vi "Main.vi"() -> ()   [LabVIEW 2018] (continued)
                    n939 = Delete From Array(array=w5529, length=2 ("长度"), index=0 ("索引")) -> (deleted portion=w5517:string[], array with subset deleted=w5526:string[])
                    n940 = call "SQL_Update.vi"("查询语句"=w5514, "表名"="Online", "error in (no error)"=w5522, "列名对应的值"=w5517, "列名"=string[] ["Last_Station", "Last_Result"], "connection reference"=w5523) -> ("error out"=w5521:errorcluster, "connection reference 2"=w5520:T5)  [unwired: 4 in]
                    n941 = call "SQL_Update.vi"("查询语句"=w5514, "表名"="Rework", "error in (no error)"=w5521, "列名对应的值"=w5526, "列名"=string[] ["ST401_Date", "ST401_Time", "ST401_Result", "ST401_PanelNumber", "ST401_Shield"], "connection reference"=w5520) -> ("error out"=w5515:errorcluster)  [unwired: 4 in, 1 out]
                    n942 = Unbundle By Name(w5515) -> ("status"=w5532:bool)
                    n943 = Equal?(x="", y=w5524) -> (x = y?=w5531:bool)
                    n944 = Or(x=w5532, y=w5531) -> (x .or. y?=w5530:bool)
                    n945 = case shown="真" w5530 {
                      tunnel: ["1" ("数据保存请求回复") "2" ("数据保存请求回复")] -> w5516
                      frame False {
                      }
                      frame True {
                      }
                    }
                  }
                }
              }
            }
            "数据保存请求回复401" <- w5445
            n946 = local write "401数据回复写入"(w5444) -> ()
            n947 = Delete From Array(array=w5433, length=2 ("长度"), index=0 ("索引")) -> (array with subset deleted=w5440:string[])  [unwired: 1 out]
            n948 = Insert Into Array(array=w5440, index=2 ("索引"), new element=w5432) -> (w5439:string[])
            n949 = Insert Into Array(array=string[][] [] ("数组"), index (row)=0 ("索引 (行)"), new element=w5439) -> (w5441:string[][])  [unwired: 1 in]
            n950 = Transpose 2D Array(2D array=w5441) -> (transposed array=w5431:string[][])
            n951 = property on="ST401_DATA" class="MCListbox (严格)"("ItemNames"=w5431) -> ()  [unwired: 2 in, 2 out]
            "ST401数据读取（事件）" <- FALSE ("ST401数据保存请求（事件）")
          }
          event "ST402扫码请求（事件）": Value Change {
            n952 = event-data() -> ()  [unwired: 1 in, 2 out]
            n953 = local read "402二维码"() -> (w5540:string)
            n954 = Concatenate Strings("Where QRCode='" ("查询语句"), w5540, "'" ("字符串")) -> (w5549:string)
            n955 = call "SQL_Select.vi"("要读取的列名"=string[] ["Last_Station", "Last_Result"], "表名"="Online", "error in (no error)"=w5541, "查询语句"=w5549, "查询条件"=TRUE, "connection reference"=w5542) -> ("error out"=w5539:errorcluster, "数据"=w5548:string[][])  [unwired: 3 in, 1 out]
            n956 = case shown="无错误" w5539 {
              tunnel: w5548 -> [w5558 _]
              tunnel: ["1" ("右扫码请求回复") "2" ("右扫码请求回复")] -> w5538
              tunnel: [TRUE TRUE] -> w5537
              frame No Error {
                n957 = Index Array(array=w5558, index (row)=0 ("索引 (行)")) -> (element=w5555:string[])  [unwired: 1 in]
                n958 = Index Array(array=w5555, index #1=0 ("索引 (行)")) -> (element #1=→"上一站号 (402)":string, element #2=→"上一站结果 (402)":string)  [unwired: 1 in]
              }
              frame Error {
              }
            }
            "扫码请求回复402" <- w5538
            n959 = local write "402扫码回复写入"(w5537) -> ()
            "ST402扫码请求（事件）" <- FALSE ("ST402扫码请求（事件）")
          }
          event "ST402数据读取（事件）": Value Change {
            w5583 = 0 ("索引 (行)")
            n960 = event-data() -> ()  [unwired: 1 in, 2 out]
            n961 = local read "402二维码"() -> (w5562:string)
            n962 = Concatenate Strings("Where QRCode='" ("查询语句"), w5562, "'" ("字符串")) -> (w5590:string)
            n963 = call "SQL_Select.vi"("要读取的列名"=string[] ["Rework_Status"], "表名"="Online", "error in (no error)"=w5576, "查询语句"=w5590, "查询条件"=TRUE, "connection reference"=w5577) -> ("error out"=w5585:errorcluster, "数据"=w5589:string[][], "connection reference out"=w5586:T5)  [unwired: 3 in]
            n964 = Index Array(array=w5589, index (row)=w5583, index (col)=w5583) -> (element=w5588:string)
            n965 = Equal?(x=w5588, y="T") -> (x = y?=w5587:bool)
            n966 = local read "402data"() -> (w5563:string[])
            n967 = case shown="真" w5587 {
              tunnel: [w5604 w5610] -> w5575
              tunnel: w5563 -> [w5603 w5613]
              tunnel: [w5598 w5609] -> w5573
              tunnel: w5562 -> [w5597 w5612]
              tunnel: w5590 -> [w5596 w5611]
              tunnel: w5586 -> [w5595 w5624]
              tunnel: w5585 -> [w5594 w5623]
              tunnel: [TRUE w5608] -> w5574
              frame False {
                n968 = call "SQL_Update.vi"("查询语句"=w5596, "表名"="Online", "error in (no error)"=w5594, "列名对应的值"=w5603, "列名"=string[] ["Last_Station", "Last_Result", "ST402_Date", "ST402_Time", "ST402_Result", "ST402_PanelNumber", "ST402_Shield"], "connection reference"=w5595) -> ("error out"=w5598:errorcluster)  [unwired: 4 in, 1 out]
                n969 = Unbundle By Name(w5598) -> ("status"=w5602:bool)
                n970 = Equal?(x=w5597, y="") -> (x = y?=w5600:bool)
                n971 = Or(x=w5602, y=w5600) -> (x .or. y?=w5599:bool)
                n972 = case shown="假" w5599 {
                  tunnel: ["1" ("数据保存请求回复") "2" ("数据保存请求回复")] -> w5604
                  frame False {
                  }
                  frame True {
                  }
                }
              }
              frame True {
                w5619 = 0 ("索引 (行)")
                n973 = call "SQL_Select.vi"("要读取的列名"=string[] ["[402]"], "表名"="Rework_List", "error in (no error)"=w5623, "查询语句"=w5611, "查询条件"=TRUE, "connection reference"=w5624) -> ("error out"=w5614:errorcluster, "数据"=w5620:string[][], "connection reference out"=w5615:T5)  [unwired: 3 in]
                n974 = Index Array(array=w5620, index (row)=w5619, index (col)=w5619) -> (element=w5618:string)
                n975 = Equal?(x=w5618, y="T") -> (x = y?=w5616:bool)
                n976 = case shown="真" w5616 {
                  tunnel: w5615 -> [w5633 w5653]
                  tunnel: w5614 -> [w5634 w5652]
                  tunnel: w5613 -> [w5632 w5659]
                  tunnel: w5612 -> [w5629 w5654]
                  tunnel: w5611 -> [w5631 w5644]
                  tunnel: [w5628 w5646] -> w5610
                  tunnel: [w5630 w5645] -> w5609
                  tunnel: [TRUE TRUE] -> w5608
                  frame False {
                    n977 = call "SQL_Update.vi"("查询语句"=w5631, "表名"="Online", "error in (no error)"=w5634, "列名对应的值"=w5632, "列名"=string[] ["Last_Station", "Last_Result", "ST402_Date", "ST402_Time", "ST402_Result", "ST402_PanelNumber", "ST402_Shield"], "connection reference"=w5633) -> ("error out"=w5630:errorcluster)  [unwired: 4 in, 1 out]
                    n978 = Unbundle By Name(w5630) -> ("status"=w5638:bool)
                    n979 = Equal?(x=w5629, y="") -> (x = y?=w5636:bool)
                    n980 = Or(x=w5638, y=w5636) -> (x .or. y?=w5635:bool)
                    n981 = case shown="假" w5635 {
                      tunnel: ["1" ("数据保存请求回复") "2" ("数据保存请求回复")] -> w5628
                      frame False {
                      }
                      frame True {
                      }
                    }
                  }
                  frame True {
                    n982 = Delete From Array(array=w5659, length=2 ("长度"), index=0 ("索引")) -> (deleted portion=w5647:string[], array with subset deleted=w5656:string[])
                    n983 = call "SQL_Update.vi"("查询语句"=w5644, "表名"="Online", "error in (no error)"=w5652, "列名对应的值"=w5647, "列名"=string[] ["Last_Station", "Last_Result"], "connection reference"=w5653) -> ("error out"=w5651:errorcluster, "connection reference 2"=w5650:T5)  [unwired: 4 in]
                    n984 = call "SQL_Update.vi"("查询语句"=w5644, "表名"="Rework", "error in (no error)"=w5651, "列名对应的值"=w5656, "列名"=string[] ["ST402_Date", "ST402_Time", "ST402_Result", "ST402_PanelNumber", "ST402_Shield"], "connection reference"=w5650) -> ("error out"=w5645:errorcluster)  [unwired: 4 in, 1 out]
                    n985 = Unbundle By Name(w5645) -> ("status"=w5662:bool)
                    n986 = Equal?(x="", y=w5654) -> (x = y?=w5661:bool)
                    n987 = Or(x=w5662, y=w5661) -> (x .or. y?=w5660:bool)
                    n988 = case shown="真" w5660 {
                      tunnel: ["1" ("数据保存请求回复") "2" ("数据保存请求回复")] -> w5646
                      frame False {
                      }
                      frame True {
                      }
                    }
                  }
                }
              }
            }
            "数据保存请求回复402" <- w5575
            n989 = local write "402数据回复写入"(w5574) -> ()
            n990 = Delete From Array(array=w5563, length=2 ("长度"), index=0 ("索引")) -> (array with subset deleted=w5570:string[])  [unwired: 1 out]
            n991 = Insert Into Array(array=w5570, index=2 ("索引"), new element=w5562) -> (w5569:string[])
            n992 = Insert Into Array(array=string[][] [] ("数组"), index (row)=0 ("索引 (行)"), new element=w5569) -> (w5571:string[][])  [unwired: 1 in]
            n993 = Transpose 2D Array(2D array=w5571) -> (transposed array=w5561:string[][])
            n994 = property on="ST402_DATA" class="MCListbox (严格)"("ItemNames"=w5561) -> ()  [unwired: 2 in, 2 out]
            "ST402数据读取（事件）" <- FALSE ("ST402数据保存请求（事件）")
          }
          event "ST501扫码请求（事件）": Value Change {
            n995 = event-data() -> ()  [unwired: 1 in, 2 out]
            n996 = local read "501二维码"() -> (w5669:string)
            n997 = Concatenate Strings("Where QRCode='" ("查询语句"), w5669, "'" ("字符串")) -> (w5679:string)
            n998 = call "SQL_Select.vi"("要读取的列名"=string[] ["Last_Station", "Last_Result"], "表名"="Online", "error in (no error)"=w5671, "查询语句"=w5679, "查询条件"=TRUE, "connection reference"=w5672) -> ("error out"=w5670:errorcluster, "数据"=w5678:string[][])  [unwired: 3 in, 1 out]
            n999 = case shown="无错误" w5670 {
              tunnel: w5678 -> [w5688 _]
              tunnel: ["1" ("右扫码请求回复") "2" ("右扫码请求回复")] -> w5668
              tunnel: [TRUE TRUE] -> w5667
              frame No Error {
                n1000 = Index Array(array=w5688, index (row)=0 ("索引 (行)")) -> (element=w5685:string[])  [unwired: 1 in]
                n1001 = Index Array(array=w5685, index #1=0 ("索引 (行)")) -> (element #1=→"上一站号 (501)":string, element #2=→"上一站结果 (501)":string)  [unwired: 1 in]
              }
              frame Error {
              }
            }
            "扫码请求回复501" <- w5668
            n1002 = local write "501扫码回复输入"(w5667) -> ()
            "ST501扫码请求（事件）" <- FALSE ("ST501扫码请求（事件）")
          }
          event "ST501数据读取（事件）": Value Change {
            w5713 = 0 ("索引 (行)")
            n1003 = event-data() -> ()  [unwired: 1 in, 2 out]
            n1004 = local read "501二维码"() -> (w5692:string)
            n1005 = Concatenate Strings("Where QRCode='" ("查询语句"), w5692, "'" ("字符串")) -> (w5720:string)
            n1006 = call "SQL_Select.vi"("要读取的列名"=string[] ["Rework_Status"], "表名"="Online", "error in (no error)"=w5706, "查询语句"=w5720, "查询条件"=TRUE, "connection reference"=w5707) -> ("error out"=w5715:errorcluster, "数据"=w5719:string[][], "connection reference out"=w5716:T5)  [unwired: 3 in]
            n1007 = Index Array(array=w5719, index (row)=w5713, index (col)=w5713) -> (element=w5718:string)
            n1008 = Equal?(x=w5718, y="T") -> (x = y?=w5717:bool)
            n1009 = local read "501data"() -> (w5693:string[])
            n1010 = case shown="真" w5717 {
              tunnel: [w5734 w5740] -> w5704
              tunnel: w5693 -> [w5733 w5743]
              tunnel: [w5728 w5739] -> w5703
              tunnel: w5692 -> [w5727 w5742]
              tunnel: w5720 -> [w5726 w5741]
              tunnel: w5716 -> [w5725 w5754]
              tunnel: w5715 -> [w5724 w5753]
              tunnel: [TRUE w5738] -> w5705
              frame False {
                n1011 = call "SQL_Update.vi"("查询语句"=w5726, "表名"="Online", "error in (no error)"=w5724, "列名对应的值"=w5733, "列名"=string[] ["Last_Station", "Last_Result", "ST501_Date", "ST501_Time", "ST501_Result", "ST501_PanelNumber", "ST501_Shield"], "connection reference"=w5725) -> ("error out"=w5728:errorcluster)  [unwired: 4 in, 1 out]
                n1012 = Unbundle By Name(w5728) -> ("status"=w5732:bool)
                n1013 = Equal?(x=w5727, y="") -> (x = y?=w5730:bool)
                n1014 = Or(x=w5732, y=w5730) -> (x .or. y?=w5729:bool)
                n1015 = case shown="假" w5729 {
                  tunnel: ["1" ("数据保存请求回复") "2" ("数据保存请求回复")] -> w5734
                  frame False {
                  }
                  frame True {
                  }
                }
              }
              frame True {
                w5749 = 0 ("索引 (行)")
                n1016 = call "SQL_Select.vi"("要读取的列名"=string[] ["[501]"], "表名"="Rework_List", "error in (no error)"=w5753, "查询语句"=w5741, "查询条件"=TRUE, "connection reference"=w5754) -> ("error out"=w5744:errorcluster, "数据"=w5750:string[][], "connection reference out"=w5745:T5)  [unwired: 3 in]
                n1017 = Index Array(array=w5750, index (row)=w5749, index (col)=w5749) -> (element=w5748:string)
                n1018 = Equal?(x=w5748, y="T") -> (x = y?=w5746:bool)
                n1019 = case shown="真" w5746 {
                  tunnel: w5745 -> [w5763 w5783]
                  tunnel: w5744 -> [w5764 w5782]
                  tunnel: w5743 -> [w5762 w5789]
                  tunnel: w5742 -> [w5759 w5784]
                  tunnel: w5741 -> [w5761 w5774]
                  tunnel: [w5758 w5776] -> w5740
                  tunnel: [w5760 w5775] -> w5739
                  tunnel: [TRUE TRUE] -> w5738
                  frame False {
                    n1020 = call "SQL_Update.vi"("查询语句"=w5761, "表名"="Online", "error in (no error)"=w5764, "列名对应的值"=w5762, "列名"=string[] ["Last_Station", "Last_Result", "ST501_Date", "ST501_Time", "ST501_Result", "ST501_PanelNumber", "ST501_Shield"], "connection reference"=w5763) -> ("error out"=w5760:errorcluster)  [unwired: 4 in, 1 out]
                    n1021 = Unbundle By Name(w5760) -> ("status"=w5768:bool)
                    n1022 = Equal?(x=w5759, y="") -> (x = y?=w5766:bool)
                    n1023 = Or(x=w5768, y=w5766) -> (x .or. y?=w5765:bool)
                    n1024 = case shown="假" w5765 {
                      tunnel: ["1" ("数据保存请求回复") "2" ("数据保存请求回复")] -> w5758
                      frame False {
                      }
                      frame True {
                      }
                    }
                  }
                  frame True {
                    n1025 = Delete From Array(array=w5789, length=2 ("长度"), index=0 ("索引")) -> (deleted portion=w5777:string[], array with subset deleted=w5786:string[])
                    n1026 = call "SQL_Update.vi"("查询语句"=w5774, "表名"="Online", "error in (no error)"=w5782, "列名对应的值"=w5777, "列名"=string[] ["Last_Station", "Last_Result"], "connection reference"=w5783) -> ("error out"=w5781:errorcluster, "connection reference 2"=w5780:T5)  [unwired: 4 in]
                    n1027 = call "SQL_Update.vi"("查询语句"=w5774, "表名"="Rework", "error in (no error)"=w5781, "列名对应的值"=w5786, "列名"=string[] ["ST501_Date", "ST501_Time", "ST501_Result", "ST501_PanelNumber", "ST501_Shield"], "connection reference"=w5780) -> ("error out"=w5775:errorcluster)  [unwired: 4 in, 1 out]
                    n1028 = Unbundle By Name(w5775) -> ("status"=w5792:bool)
                    n1029 = Equal?(x="", y=w5784) -> (x = y?=w5791:bool)
                    n1030 = Or(x=w5792, y=w5791) -> (x .or. y?=w5790:bool)
                    n1031 = case shown="真" w5790 {
                      tunnel: ["1" ("数据保存请求回复") "2" ("数据保存请求回复")] -> w5776
                      frame False {
                      }
                      frame True {
                      }
                    }
                  }
                }
              }
            }
            "数据保存请求回复501" <- w5704
            n1032 = local write "501数据回复输入"(w5705) -> ()
            n1033 = Delete From Array(array=w5693, length=2 ("长度"), index=0 ("索引")) -> (array with subset deleted=w5700:string[])  [unwired: 1 out]
            n1034 = Insert Into Array(array=w5700, index=2 ("索引"), new element=w5692) -> (w5699:string[])
            n1035 = Insert Into Array(array=string[][] [] ("数组"), index (row)=0 ("索引 (行)"), new element=w5699) -> (w5701:string[][])  [unwired: 1 in]
            n1036 = Transpose 2D Array(2D array=w5701) -> (transposed array=w5691:string[][])
            n1037 = property on="ST501_DATA" class="MCListbox (严格)"("ItemNames"=w5691) -> ()  [unwired: 2 in, 2 out]
            "ST501数据读取（事件）" <- FALSE ("ST501数据读取（事件）")
          }
          event "ST502扫码请求（事件）": Value Change {
            w5797 = path "D:/op50" ("路径")
            n1038 = event-data() -> ()  [unwired: 1 in, 2 out]
            n1039 = List Folder(path=w5797) -> (filenames=w5796:string[])  [unwired: 3 in, 3 out]
            n1040 = for {
              tunnel: w5796 -> [w5815] mode=indexing
              tunnel: w5797 -> [w5816]
              n1041 = Build Path(base path=w5816, name or relative path=w5815) -> (appended path=w5813:path)
              n1042 = Delete(path (use dialog)=w5813, entire hierarchy (F)=TRUE ("整个层次结构(F)")) -> ()  [unwired: 3 in, 3 out]
            }
            n1043 = local read "502二维码"() -> (w5802:string)
            n1044 = Concatenate Strings("Where QRCode='" ("查询语句"), w5802, "'" ("字符串")) -> (w5811:string)
            n1045 = call "SQL_Select.vi"("要读取的列名"=string[] ["Last_Station", "Last_Result"], "表名"="Online", "error in (no error)"=w5803, "查询语句"=w5811, "查询条件"=TRUE, "connection reference"=w5804) -> ("error out"=w5801:errorcluster, "数据"=w5810:string[][])  [unwired: 3 in, 1 out]
            n1046 = case shown="无错误" w5801 {
              tunnel: w5810 -> [w5824 _]
              tunnel: ["1" ("右扫码请求回复") "2" ("右扫码请求回复")] -> w5800
              tunnel: [TRUE TRUE] -> w5799
              frame No Error {
                n1047 = Index Array(array=w5824, index (row)=0 ("索引 (行)")) -> (element=w5821:string[])  [unwired: 1 in]
                n1048 = Index Array(array=w5821, index #1=0 ("索引 (行)")) -> (element #1=→"上一站号 (502)":string, element #2=→"上一站结果 (502)":string)  [unwired: 1 in]
              }
              frame Error {
              }
            }
            "扫码请求回复502" <- w5800
            n1049 = local write "502扫码回复输入"(w5799) -> ()
            "ST502扫码请求（事件）" <- FALSE ("ST502扫码请求（事件）")
          }
          event "ST502数据读取（事件）": Value Change {
            w5848 = 0 ("索引 (行)")
            n1050 = event-data() -> ()  [unwired: 1 in, 2 out]
            n1051 = local read "502二维码"() -> (w5829:string)
            n1052 = Concatenate Strings("Where QRCode='" ("查询语句"), w5829, "'" ("字符串")) -> (w5855:string)
            n1053 = call "SQL_Select.vi"("要读取的列名"=string[] ["Rework_Status"], "表名"="Online", "error in (no error)"=w5842, "查询语句"=w5855, "查询条件"=TRUE, "connection reference"=w5841) -> ("error out"=w5850:errorcluster, "数据"=w5854:string[][], "connection reference out"=w5851:T5)  [unwired: 3 in]
            n1054 = Index Array(array=w5854, index (row)=w5848, index (col)=w5848) -> (element=w5853:string)
            n1055 = Equal?(x=w5853, y="T") -> (x = y?=w5852:bool)
            n1056 = local read "502数据"() -> (w5830:string[])
            n1057 = case shown="真" w5852 {
              tunnel: w5830 -> [w5870 w5878]
              tunnel: [w5866 w5875] -> w5840
              tunnel: w5829 -> [w5865 w5877]
              tunnel: w5855 -> [w5864 w5876]
              tunnel: w5851 -> [w5863 w5889]
              tunnel: w5850 -> [w5862 w5888]
              tunnel: [w5860 w5874] -> w5827
              frame False {
                n1058 = call "SQL_Update.vi"("查询语句"=w5864, "表名"="Online", "error in (no error)"=w5862, "列名对应的值"=w5870, "列名"=string[] ["Last_Station", "Last_Result", "ST502_Date", "ST502_Time", "ST502_Result", "ST502_PanelNumber", "ST502_Pressure_Final1", "ST502_Distance_Final1", "ST502_Pressure_Upper1", "ST502_Pressure_Lower1", "ST502_Distance_Upper1", "ST502_Distance_Lower1", "ST502_Pressure_Final2", "ST502_Distance_Final2", "ST502_Pressure_Upper2", "ST502_Pressure_Lower2", "ST502_Distance_Upper2", "ST502_Distance_Lower2", "ST502_Inflexion_force_Left_Final", "ST502_Inflexion_force_Left_Upper", "ST502_Inflexion_force_Left_Lower", "ST502_Inflexion_force_Right_Final", "ST502_Inflexion_force_Right_Upper", "ST502_Inflexion_force_Right_Lower"], "connection reference"=w5863) -> ("error out"=w5866:errorcluster)  [unwired: 4 in, 1 out]
                n1059 = Unbundle By Name(w5866) -> ("status"=w5869:bool)
                n1060 = Equal?(x=w5865, y="") -> (x = y?=w5867:bool)
                n1061 = Or(x=w5869, y=w5867) -> (x .or. y?=w5860:bool)
                n1062 = case shown="假" w5860 {
                  tunnel: ["1" ("数据保存请求回复") "2" ("数据保存请求回复")] -> _
                  frame False {
                  }
                  frame True {
                  }
                }
              }
              frame True {
                w5884 = 0 ("索引 (行)")
                n1063 = call "SQL_Select.vi"("要读取的列名"=string[] ["[502]"], "表名"="Rework_List", "error in (no error)"=w5888, "查询语句"=w5876, "查询条件"=TRUE, "connection reference"=w5889) -> ("error out"=w5879:errorcluster, "数据"=w5885:string[][], "connection reference out"=w5880:T5)  [unwired: 3 in]
                n1064 = Index Array(array=w5885, index (row)=w5884, index (col)=w5884) -> (element=w5883:string)
                n1065 = Equal?(x=w5883, y="T") -> (x = y?=w5881:bool)
                n1066 = case shown="假" w5881 {
                  tunnel: w5880 -> [w5897 w5915]
                  tunnel: w5879 -> [w5898 w5914]
                  tunnel: w5878 -> [w5896 w5921]
                  tunnel: w5877 -> [w5893 w5916]
                  tunnel: w5876 -> [w5895 w5907]
                  tunnel: [w5894 w5908] -> w5875
                  tunnel: [w5891 w5905] -> w5874
                  frame False {
                    (unwired) TRUE
                    n1067 = call "SQL_Update.vi"("查询语句"=w5895, "表名"="Online", "error in (no error)"=w5898, "列名对应的值"=w5896, "列名"=string[] ["Last_Station", "Last_Result", "ST502_Date", "ST502_Time", "ST502_Result", "ST502_PanelNumber", "ST502_Pressure_Final1", "ST502_Distance_Final1", "ST502_Pressure_Upper1", "ST502_Pressure_Lower1", "ST502_Distance_Upper1", "ST502_Distance_Lower1", "ST502_Pressure_Final2", "ST502_Distance_Final2", "ST502_Pressure_Upper2", "ST502_Pressure_Lower2", "ST502_Distance_Upper2", "ST502_Distance_Lower2", "ST502_Inflexion_force_Left_Final", "ST502_Inflexion_force_Left_Upper", "ST502_Inflexion_force_Left_Lower", "ST502_Inflexion_force_Right_Final", "ST502_Inflexion_force_Right_Upper", "ST502_Inflexion_force_Right_Lower"], "connection reference"=w5897) -> ("error out"=w5894:errorcluster)  [unwired: 4 in, 1 out]
                    n1068 = Unbundle By Name(w5894) -> ("status"=w5901:bool)
                    n1069 = Equal?(x=w5893, y="") -> (x = y?=w5899:bool)
                    n1070 = Or(x=w5901, y=w5899) -> (x .or. y?=w5891:bool)
                    n1071 = case shown="假" w5891 {
                      tunnel: ["1" ("数据保存请求回复") "2" ("数据保存请求回复")] -> _
                      frame False {
                      }
                      frame True {
                      }
                    }
                  }
                  frame True {
                    n1072 = Delete From Array(array=w5921, length=2 ("长度"), index=0 ("索引")) -> (deleted portion=w5909:string[], array with subset deleted=w5918:string[])
                    n1073 = call "SQL_Update.vi"("查询语句"=w5907, "表名"="Online", "error in (no error)"=w5914, "列名对应的值"=w5909, "列名"=string[] ["Last_Station", "Last_Result"], "connection reference"=w5915) -> ("error out"=w5913:errorcluster, "connection reference 2"=w5912:T5)  [unwired: 4 in]
                    n1074 = call "SQL_Update.vi"("查询语句"=w5907, "表名"="Rework", "error in (no error)"=w5913, "列名对应的值"=w5918, "列名"=string[] ["ST502_Date", "ST502_Time", "ST502_Result", "ST502_PanelNumber", "ST502_Pressure_Final1", "ST502_Distance_Final1", "ST502_Pressure_Upper1", "ST502_Pressure_Lower1", "ST502_Distance_Upper1", "ST502_Distance_Lower1", "ST502_Pressure_Final2", "ST502_Distance_Final2", "ST502_Pressure_Upper2", "ST502_Pressure_Lower2", "ST502_Distance_Upper2", "ST502_Distance_Lower2", "ST502_Inflexion_force_Left_Final", "ST502_Inflexion_force_Left_Upper", "ST502_Inflexion_force_Left_Lower", "ST502_Inflexion_force_Right_Final", "ST502_Inflexion_force_Right_Upper", "ST502_Inflexion_force_Right_Lower"], "connection reference"=w5912) -> ("error out"=w5908:errorcluster)  [unwired: 4 in, 1 out]
                    n1075 = Unbundle By Name(w5908) -> ("status"=w5923:bool)
                    n1076 = Equal?(x="", y=w5916) -> (x = y?=w5922:bool)
                    n1077 = Or(x=w5923, y=w5922) -> (x .or. y?=w5905:bool)
                    n1078 = case shown="真" w5905 {
                      tunnel: ["1" ("数据保存请求回复") "2" ("数据保存请求回复")] -> _
                      frame False {
                      }
                      frame True {
                      }
                    }
                  }
                }
              }
            }
            n1079 = Delete From Array(array=w5830, length=2 ("长度"), index=0 ("索引")) -> (array with subset deleted=w5837:string[])  [unwired: 1 out]
            n1080 = Insert Into Array(array=w5837, index=2 ("索引"), new element=w5829) -> (w5836:string[])
            n1081 = Insert Into Array(array=string[][] [] ("数组"), index (row)=0 ("索引 (行)"), new element=w5836) -> (w5838:string[][])  [unwired: 1 in]
            n1082 = case shown="假" w5827 {
              frame False {
                n1083 = property on="ST502画曲线" class="Bool (严格)"("Val(Sgnl)"=TRUE ("值(信号)")) -> ()  [unwired: 2 in, 2 out]
              }
              frame True {
                n1084 = local write "502数据回复输入"(TRUE ("502数据回复输入")) -> ()
                "数据保存请求回复502" <- "2" ("数据保存请求回复502")
              }
            }
            n1085 = Transpose 2D Array(2D array=w5838) -> (transposed array=w5828:string[][])
            n1086 = property on="ST502_DATA" class="MCListbox (严格)"("ItemNames"=w5828) -> ()  [unwired: 2 in, 2 out]
            "ST502数据读取（事件）" <- FALSE ("ST502数据读取（事件）")
          }
          event "ST503扫码请求（事件）": Value Change {
            n1087 = event-data() -> ()  [unwired: 1 in, 2 out]
            n1088 = local read "503二维码"() -> (w5930:string)
            n1089 = Concatenate Strings("Where QRCode='" ("查询语句"), w5930, "'" ("字符串")) -> (w5940:string)
            n1090 = call "SQL_Select.vi"("要读取的列名"=string[] ["Last_Station", "Last_Result"], "表名"="Online", "error in (no error)"=w5933, "查询语句"=w5940, "查询条件"=TRUE, "connection reference"=w5934) -> ("error out"=w5932:errorcluster, "数据"=w5939:string[][])  [unwired: 3 in, 1 out]
            n1091 = case shown="无错误" w5932 {
              tunnel: w5939 -> [w5949 _]
              tunnel: ["1" ("右扫码请求回复") "2" ("右扫码请求回复")] -> w5928
              tunnel: [TRUE TRUE] -> w5927
              frame No Error {
                n1092 = Index Array(array=w5949, index (row)=0 ("索引 (行)")) -> (element=w5946:string[])  [unwired: 1 in]
                n1093 = Index Array(array=w5946, index #1=0 ("索引 (行)")) -> (element #1=→"上一站号 (503)":string, element #2=→"上一站结果 (503)":string)  [unwired: 1 in]
              }
              frame Error {
              }
            }
            "扫码请求回复503" <- w5928
            n1094 = local write "503扫码回复输入"(w5927) -> ()
            "ST503扫码请求（事件）" <- FALSE ("ST503扫码请求（事件）")
          }
          event "ST503数据读取（事件）": Value Change {
            w5974 = 0 ("索引 (行)")
            n1095 = event-data() -> ()  [unwired: 1 in, 2 out]
            n1096 = local read "503二维码"() -> (w5953:string)
            n1097 = Concatenate Strings("Where QRCode='" ("查询语句"), w5953, "'" ("字符串")) -> (w5981:string)
            n1098 = call "SQL_Select.vi"("要读取的列名"=string[] ["Rework_Status"], "表名"="Online", "error in (no error)"=w5968, "查询语句"=w5981, "查询条件"=TRUE, "connection reference"=w5967) -> ("error out"=w5976:errorcluster, "数据"=w5980:string[][], "connection reference out"=w5977:T5)  [unwired: 3 in]
            n1099 = Index Array(array=w5980, index (row)=w5974, index (col)=w5974) -> (element=w5979:string)
            n1100 = Equal?(x=w5979, y="T") -> (x = y?=w5978:bool)
            n1101 = local read "503data"() -> (w5954:string[])
            n1102 = case shown="假" w5978 {
              tunnel: [w5995 w6001] -> w5963
              tunnel: w5954 -> [w5994 w6004]
              tunnel: [w5989 w6000] -> w5966
              tunnel: w5953 -> [w5988 w6003]
              tunnel: w5981 -> [w5987 w6002]
              tunnel: w5977 -> [w5986 w6015]
              tunnel: w5976 -> [w5985 w6014]
              tunnel: [TRUE w5999] -> w5964
              frame False {
                n1103 = call "SQL_Update.vi"("查询语句"=w5987, "表名"="Online", "error in (no error)"=w5985, "列名对应的值"=w5994, "列名"=string[] ["Last_Station", "Last_Result", "ST503_Date", "ST503_Time", "ST503_Result", "ST503_PanelNumber", "ST503_Pin", "ST503_Position_degree"], "connection reference"=w5986) -> ("error out"=w5989:errorcluster)  [unwired: 4 in, 1 out]
                n1104 = Unbundle By Name(w5989) -> ("status"=w5993:bool)
                n1105 = Equal?(x=w5988, y="") -> (x = y?=w5991:bool)
                n1106 = Or(x=w5993, y=w5991) -> (x .or. y?=w5990:bool)
                n1107 = case shown="真" w5990 {
                  tunnel: ["1" ("数据保存请求回复") "2" ("数据保存请求回复")] -> w5995
                  frame False {
                  }
                  frame True {
                  }
                }
              }
              frame True {
                w6010 = 0 ("索引 (行)")
                n1108 = call "SQL_Select.vi"("要读取的列名"=string[] ["[503]"], "表名"="Rework_List", "error in (no error)"=w6014, "查询语句"=w6002, "查询条件"=TRUE, "connection reference"=w6015) -> ("error out"=w6005:errorcluster, "数据"=w6011:string[][], "connection reference out"=w6006:T5)  [unwired: 3 in]
                n1109 = Index Array(array=w6011, index (row)=w6010, index (col)=w6010) -> (element=w6009:string)
                n1110 = Equal?(x=w6009, y="T") -> (x = y?=w6007:bool)
                n1111 = case shown="真" w6007 {
                  tunnel: w6006 -> [w6024 w6044]
                  tunnel: w6005 -> [w6025 w6043]
                  tunnel: w6004 -> [w6023 w6050]
                  tunnel: w6003 -> [w6020 w6045]
                  tunnel: w6002 -> [w6022 w6035]
                  tunnel: [w6019 w6037] -> w6001
                  tunnel: [w6021 w6036] -> w6000
                  tunnel: [TRUE TRUE] -> w5999
                  frame False {
                    n1112 = call "SQL_Update.vi"("查询语句"=w6022, "表名"="Online", "error in (no error)"=w6025, "列名对应的值"=w6023, "列名"=string[] ["Last_Station", "Last_Result", "ST503_Date", "ST503_Time", "ST503_Result", "ST503_PanelNumber", "ST503_Pin", "ST503_Position_degree"], "connection reference"=w6024) -> ("error out"=w6021:errorcluster)  [unwired: 4 in, 1 out]
                    n1113 = Unbundle By Name(w6021) -> ("status"=w6029:bool)
                    n1114 = Equal?(x=w6020, y="") -> (x = y?=w6027:bool)
                    n1115 = Or(x=w6029, y=w6027) -> (x .or. y?=w6026:bool)
                    n1116 = case shown="假" w6026 {
                      tunnel: ["1" ("数据保存请求回复") "2" ("数据保存请求回复")] -> w6019
                      frame False {
                      }
                      frame True {
                      }
                    }
                  }
                  frame True {
                    n1117 = Delete From Array(array=w6050, length=2 ("长度"), index=0 ("索引")) -> (deleted portion=w6038:string[], array with subset deleted=w6047:string[])
                    n1118 = call "SQL_Update.vi"("查询语句"=w6035, "表名"="Online", "error in (no error)"=w6043, "列名对应的值"=w6038, "列名"=string[] ["Last_Station", "Last_Result"], "connection reference"=w6044) -> ("error out"=w6042:errorcluster, "connection reference 2"=w6041:T5)  [unwired: 4 in]
                    n1119 = call "SQL_Update.vi"("查询语句"=w6035, "表名"="Rework", "error in (no error)"=w6042, "列名对应的值"=w6047, "列名"=string[] ["ST503_Date", "ST503_Time", "ST503_Result", "ST503_PanelNumber", "ST503_Pin", "ST503_Position_degree"], "connection reference"=w6041) -> ("error out"=w6036:errorcluster)  [unwired: 4 in, 1 out]
                    n1120 = Unbundle By Name(w6036) -> ("status"=w6053:bool)
                    n1121 = Equal?(x="", y=w6045) -> (x = y?=w6052:bool)
                    n1122 = Or(x=w6053, y=w6052) -> (x .or. y?=w6051:bool)
                    n1123 = case shown="真" w6051 {
                      tunnel: ["1" ("数据保存请求回复") "2" ("数据保存请求回复")] -> w6037
                      frame False {
                      }
                      frame True {
                      }
                    }
                  }
                }
              }
            }
            "数据保存请求回复503" <- w5963
            n1124 = local write "503数据回复输入"(w5964) -> ()
            n1125 = Delete From Array(array=w5954, length=2 ("长度"), index=0 ("索引")) -> (array with subset deleted=w5961:string[])  [unwired: 1 out]
            n1126 = Insert Into Array(array=w5961, index=2 ("索引"), new element=w5953) -> (w5960:string[])
            n1127 = Insert Into Array(array=string[][] [] ("数组"), index (row)=0 ("索引 (行)"), new element=w5960) -> (w5962:string[][])  [unwired: 1 in]
            n1128 = Transpose 2D Array(2D array=w5962) -> (transposed array=w5952:string[][])
            n1129 = property on="ST503_DATA" class="MCListbox (严格)"("ItemNames"=w5952) -> ()  [unwired: 2 in, 2 out]
            "ST503数据读取（事件）" <- FALSE ("ST503数据读取（事件）")
          }
          event "ST504扫码请求（事件）": Value Change {
            n1130 = event-data() -> ()  [unwired: 1 in, 2 out]
            n1131 = local read "504二维码"() -> (w6061:string)
            n1132 = Concatenate Strings("Where QRCode='" ("查询语句"), w6061, "'" ("字符串")) -> (w6070:string)
            n1133 = call "SQL_Select.vi"("要读取的列名"=string[] ["Last_Station", "Last_Result"], "表名"="Online", "error in (no error)"=w6062, "查询语句"=w6070, "查询条件"=TRUE, "connection reference"=w6063) -> ("error out"=w6060:errorcluster, "数据"=w6069:string[][])  [unwired: 3 in, 1 out]
            n1134 = case shown="无错误" w6060 {
              tunnel: w6069 -> [w6079 _]
              tunnel: ["1" ("右扫码请求回复") "2" ("右扫码请求回复")] -> w6058
              tunnel: [TRUE TRUE] -> w6057
              frame No Error {
                n1135 = Index Array(array=w6079, index (row)=0 ("索引 (行)")) -> (element=w6076:string[])  [unwired: 1 in]
                n1136 = Index Array(array=w6076, index #1=0 ("索引 (行)")) -> (element #1=→"上一站号 (504)":string, element #2=→"上一站结果 (504)":string)  [unwired: 1 in]
              }
              frame Error {
              }
            }
            "扫码请求回复504" <- w6058
            n1137 = local write "504扫码回复输入"(w6057) -> ()
            "ST504扫码请求（事件）" <- FALSE ("ST504扫码请求（事件）")
          }
          event "ST504数据读取（事件）": Value Change {
            n1138 = event-data() -> ()  [unwired: 1 in, 2 out]
            n1139 = local read "504二维码"() -> (w6083:string)
            n1140 = Not Equal?(x=w6083, y="") -> (x != y?=w6087:bool)
            n1141 = Concatenate Strings("Where QRCode='" ("查询语句"), w6083, "'" ("字符串")) -> (w6084:string)
            n1142 = case shown="真" w6087 {
              tunnel: w6092 -> [_ w6123]
              tunnel: w6091 -> [_ w6122]
              tunnel: [errorcluster {"status"=TRUE, "code"=0, "source"="，二维码为空"} ("error out") w6103] -> w6090
              tunnel: w6083 -> [_ w6113]
              tunnel: w6084 -> [_ w6107]
              tunnel: ["2" ("数据保存请求回复") w6102] -> w6082
              frame False {
              }
              frame True {
                w6127 = 0 ("索引 (行)")
                n1143 = local read "504data"() -> (w6108:string[])
                n1144 = call "SQL_Select.vi"("要读取的列名"=string[] ["Rework_Status"], "表名"="Online", "error in (no error)"=w6122, "查询语句"=w6107, "查询条件"=TRUE, "connection reference"=w6123) -> ("error out"=w6104:errorcluster, "数据"=w6130:string[][], "connection reference out"=w6105:T5)  [unwired: 3 in]
                n1145 = Index Array(array=w6130, index (row)=w6127, index (col)=w6127) -> (element=w6129:string)
                n1146 = Equal?(x=w6129, y="T") -> (x = y?=w6106:bool)
                n1147 = flat-sequence {
                  tunnel: w6105 -> [w6141]
                  tunnel: w6104 -> [w6140]
                  tunnel: w6108 -> [w6139]
                  tunnel: w6107 -> [w6138]
                  tunnel: [w6137] -> w6111
                  tunnel: [w6136] -> w6110
                  tunnel: [w6135] -> w6109
                  tunnel: w6106 -> [w6134]
                  tunnel: [w6134] -> w6101
                  tunnel: [w6133] -> w6100
                  tunnel: [w6132] -> w6099
                  tunnel: [w6131] -> w6098
                  tunnel: w6111 -> [w6201]
                  tunnel: w6110 -> [w6209]
                  tunnel: [w6202] -> w6102
                  tunnel: w6109 -> [w6200]
                  tunnel: [w6194] -> w6103
                  tunnel: w6101 -> [w6199]
                  tunnel: w6100 -> [w6196]
                  tunnel: w6099 -> [w6195]
                  tunnel: w6098 -> [w6193]
                  frame #0 {
                    n1148 = case shown="假" w6134 {
                      tunnel: w6139 -> [w6143 w6153]
                      tunnel: [w6149 w6156] -> w6135
                      tunnel: w6138 -> [w6144 w6157]
                      tunnel: w6141 -> [w6148 w6167]
                      tunnel: w6140 -> [w6147 w6166]
                      tunnel: [w6145 w6155] -> w6137
                      tunnel: [w6144 w6154] -> w6136
                      tunnel: [w6144 w6152] -> w6133
                      tunnel: [w6143 w6153] -> w6132
                      tunnel: [FALSE w6151] -> w6131
                      frame False {
                        n1149 = call "SQL_Update.vi"("查询语句"=w6144, "表名"="Online", "error in (no error)"=w6147, "列名对应的值"=w6143, "列名"=string[] ["Last_Station", "Last_Result", "ST504_Date", "ST504_Time", "ST504_Result", "ST504_PanelNumber", "ST504_Small_Sealing_Ring_Exit", "ST504_Big_Sealing_Ring_Exit", "ST504_Big_Sealing_Ring_Number", "ST504_Small_Sealing_Ring_Excess", "ST504_Retaining_Ring_LH2110811", "ST504_Pressure_Plate_5020472", "ST504_O_ring_5003059", "ST504_O_ring_5003061", "ST504_Spring_Dowel_Pin_5018182"], "connection reference"=w6148) -> ("error out"=w6149:errorcluster, "connection reference 2"=w6145:T5)  [unwired: 4 in]
                      }
                      frame True {
                        w6162 = 0 ("索引 (行)")
                        n1150 = call "SQL_Select.vi"("要读取的列名"=string[] ["[504]"], "表名"="Rework_List", "error in (no error)"=w6166, "查询语句"=w6157, "查询条件"=TRUE, "connection reference"=w6167) -> ("error out"=w6158:errorcluster, "数据"=w6163:string[][], "connection reference out"=w6159:T5)  [unwired: 3 in]
                        n1151 = Index Array(array=w6163, index (row)=w6162, index (col)=w6162) -> (element=w6161:string)
                        n1152 = Equal?(x=w6161, y="T") -> (x = y?=w6151:bool)
                        n1153 = case shown="真" w6151 {
                          tunnel: w6159 -> [w6174 w6187]
                          tunnel: w6158 -> [w6175 w6186]
                          tunnel: w6153 -> [w6173 w6191]
                          tunnel: w6157 -> [w6169 w6177]
                          tunnel: [w6172 w6180] -> w6156
                          tunnel: [w6170 w6178] -> w6155
                          tunnel: [w6169 w6177] -> w6154
                          tunnel: [w6169 w6177] -> w6152
                          frame False {
                            n1154 = call "SQL_Update.vi"("查询语句"=w6169, "表名"="Online", "error in (no error)"=w6175, "列名对应的值"=w6173, "列名"=string[] ["Last_Station", "Last_Result", "ST504_Date", "ST504_Time", "ST504_Result", "ST504_PanelNumber", "ST504_Small_Sealing_Ring_Exit", "ST504_Big_Sealing_Ring_Exit", "ST504_Big_Sealing_Ring_Number", "ST504_Small_Sealing_Ring_Excess", "ST504_Retaining_Ring_LH2110811", "ST504_Pressure_Plate_5020472", "ST504_O_ring_5003059", "ST504_O_ring_5003061", "ST504_Spring_Dowel_Pin_5018182"], "connection reference"=w6174) -> ("error out"=w6172:errorcluster, "connection reference 2"=w6170:T5)  [unwired: 4 in]
                          }
                          frame True {
                            n1155 = Delete From Array(array=w6191, length=2 ("长度"), index=0 ("索引")) -> (deleted portion=w6181:string[], array with subset deleted=w6188:string[])
                            n1156 = call "SQL_Update.vi"("查询语句"=w6177, "表名"="Online", "error in (no error)"=w6186, "列名对应的值"=w6181, "列名"=string[] ["Last_Station", "Last_Result"], "connection reference"=w6187) -> ("error out"=w6185:errorcluster, "connection reference 2"=w6184:T5)  [unwired: 4 in]
                            n1157 = call "SQL_Update.vi"("查询语句"=w6177, "表名"="Rework", "error in (no error)"=w6185, "列名对应的值"=w6188, "列名"=string[] ["ST504_Date", "ST504_Time", "ST504_Result", "ST504_PanelNumber", "ST504_Small_Sealing_Ring_Exit", "ST504_Big_Sealing_Ring_Exit", "ST504_Big_Sealing_Ring_Number", "ST504_Small_Sealing_Ring_Excess", "ST504_Retaining_Ring_LH2110811", "ST504_Pressure_Plate_5020472", "ST504_O_ring_5003059", "ST504_O_ring_5003061", "ST504_Spring_Dowel_Pin_5018182"], "connection reference"=w6184) -> ("error out"=w6180:errorcluster, "connection reference 2"=w6178:T5)  [unwired: 4 in]
                          }
                        }
                      }
                    }
                  }
                  frame #1 {
                    w6203 = 0 ("索引 (行)")
                    n1158 = call "SQL_Select.vi"("要读取的列名"=string[] ["Last_Station"], "表名"="Online", "error in (no error)"=w6200, "查询语句"=w6209, "查询条件"=TRUE, "connection reference"=w6201) -> ("error out"=w6197:errorcluster, "数据"=w6204:string[][], "connection reference out"=w6198:T5)  [unwired: 3 in]
                    n1159 = Index Array(array=w6204, index (row)=w6203) -> (element=w6208:string[])  [unwired: 1 in]
                    n1160 = Index Array(array=w6208, index=w6203) -> (element=w6207:string)
                    n1161 = Equal?(x=w6207, y="504") -> (x = y?=w6205:bool)
                    n1162 = case shown="假" w6205 {
                      tunnel: [w6214 "1"] -> w6202
                      tunnel: w6199 -> [w6234 _]
                      tunnel: w6198 -> [w6233 _]
                      tunnel: w6197 -> [w6232 w6275]
                      tunnel: w6196 -> [w6231 _]
                      tunnel: w6195 -> [w6230 _]
                      tunnel: [w6219 w6275] -> w6194
                      tunnel: w6193 -> [w6213 _]
                      frame False {
                        w6223 = 0 ("索引 (行)")
                        n1163 = case shown="真" w6234 {
                          tunnel: w6233 -> [w6240 w6250]
                          tunnel: w6232 -> [w6239 w6249]
                          tunnel: w6231 -> [w6235 w6247]
                          tunnel: w6230 -> [w6238 w6248]
                          tunnel: [w6237 w6246] -> w6221
                          tunnel: [w6236 w6245] -> w6220
                          tunnel: [w6235 w6244] -> w6222
                          tunnel: w6213 -> [_ w6243]
                          frame False {
                            n1164 = call "SQL_Update.vi"("查询语句"=w6235, "表名"="Online", "error in (no error)"=w6239, "列名对应的值"=w6238, "列名"=string[] ["Last_Station", "Last_Result", "ST504_Date", "ST504_Time", "ST504_Result", "ST504_PanelNumber", "ST504_Small_Sealing_Ring_Exit", "ST504_Big_Sealing_Ring_Exit", "ST504_Big_Sealing_Ring_Number", "ST504_Small_Sealing_Ring_Excess", "ST504_Retaining_Ring_LH2110811", "ST504_Pressure_Plate_5020472", "ST504_O_ring_5003059", "ST504_O_ring_5003061", "ST504_Spring_Dowel_Pin_5018182"], "connection reference"=w6240) -> ("error out"=w6237:errorcluster, "connection reference 2"=w6236:T5)  [unwired: 4 in]
                          }
                          frame True {
                            n1165 = case shown="真" w6243 {
                              tunnel: w6250 -> [w6256 w6269]
                              tunnel: w6249 -> [w6257 w6268]
                              tunnel: w6248 -> [w6255 w6273]
                              tunnel: w6247 -> [w6251 w6259]
                              tunnel: [w6254 w6262] -> w6246
                              tunnel: [w6252 w6260] -> w6245
                              tunnel: [w6251 w6259] -> w6244
                              frame False {
                                n1166 = call "SQL_Update.vi"("查询语句"=w6251, "表名"="Online", "error in (no error)"=w6257, "列名对应的值"=w6255, "列名"=string[] ["Last_Station", "Last_Result", "ST504_Date", "ST504_Time", "ST504_Result", "ST504_PanelNumber", "ST504_Small_Sealing_Ring_Exit", "ST504_Big_Sealing_Ring_Exit", "ST504_Big_Sealing_Ring_Number", "ST504_Small_Sealing_Ring_Excess", "ST504_Retaining_Ring_LH2110811", "ST504_Pressure_Plate_5020472", "ST504_O_ring_5003059", "ST504_O_ring_5003061", "ST504_Spring_Dowel_Pin_5018182"], "connection reference"=w6256) -> ("error out"=w6254:errorcluster, "connection reference 2"=w6252:T5)  [unwired: 4 in]
                              }
                              frame True {
                                n1167 = Delete From Array(array=w6273, length=2 ("长度"), index=0 ("索引")) -> (deleted portion=w6263:string[], array with subset deleted=w6270:string[])
                                n1168 = call "SQL_Update.vi"("查询语句"=w6259, "表名"="Online", "error in (no error)"=w6268, "列名对应的值"=w6263, "列名"=string[] ["Last_Station", "Last_Result"], "connection reference"=w6269) -> ("error out"=w6267:errorcluster, "connection reference 2"=w6266:T5)  [unwired: 4 in]
                                n1169 = call "SQL_Update.vi"("查询语句"=w6259, "表名"="Rework", "error in (no error)"=w6267, "列名对应的值"=w6270, "列名"=string[] ["ST504_Date", "ST504_Time", "ST504_Result", "ST504_PanelNumber", "ST504_Small_Sealing_Ring_Exit", "ST504_Big_Sealing_Ring_Exit", "ST504_Big_Sealing_Ring_Number", "ST504_Small_Sealing_Ring_Excess", "ST504_Retaining_Ring_LH2110811", "ST504_Pressure_Plate_5020472", "ST504_O_ring_5003059", "ST504_O_ring_5003061", "ST504_Spring_Dowel_Pin_5018182"], "connection reference"=w6266) -> ("error out"=w6262:errorcluster, "connection reference 2"=w6260:T5)  [unwired: 4 in]
                              }
                            }
                          }
                        }
                        n1170 = call "SQL_Select.vi"("要读取的列名"=string[] ["Last_Station"], "表名"="Online", "error in (no error)"=w6221, "查询语句"=w6222, "查询条件"=TRUE, "connection reference"=w6220) -> ("error out"=w6219:errorcluster, "数据"=w6224:string[][])  [unwired: 3 in, 1 out]
                        n1171 = Index Array(array=w6224, index (row)=w6223) -> (element=w6227:string[])  [unwired: 1 in]
                        n1172 = Index Array(array=w6227, index=w6223) -> (element=w6226:string)
                        n1173 = Equal?(x=w6226, y="504") -> (x = y?=w6217:bool)
                        n1174 = Select(t="1", s=w6217, f="2") -> (s? t:f=w6214:string)
                      }
                      frame True {
                      }
                    }
                  }
                }
                n1175 = Delete From Array(array=w6108, length=2 ("长度"), index=0 ("索引")) -> (array with subset deleted=w6120:string[])  [unwired: 1 out]
                n1176 = Insert Into Array(array=w6120, index=2 ("索引"), new element=w6113) -> (w6119:string[])
                n1177 = Insert Into Array(array=string[][] [] ("数组"), index (row)=0 ("索引 (行)"), new element=w6119) -> (w6121:string[][])  [unwired: 1 in]
                n1178 = Transpose 2D Array(2D array=w6121) -> (transposed array=w6112:string[][])
                n1179 = property on="ST504_DATA" class="MCListbox (严格)"("ItemNames"=w6112) -> ()  [unwired: 2 in, 2 out]
              }
            }
            n1180 = flat-sequence {
              tunnel: w6082 -> [w6094]
              frame #0 {
                "数据保存请求回复504" <- w6094
              }
              frame #1 {
                n1181 = local write "504数据回复输入"(TRUE) -> ()
              }
            }
            "ST504数据读取（事件）" <- FALSE ("ST504数据读取（事件）")
          }
          event "ST601扫码请求（事件）": Value Change {
            n1182 = event-data() -> ()  [unwired: 1 in, 2 out]
            n1183 = local read "601二维码"() -> (w6283:string)
            n1184 = Concatenate Strings("Where QRCode='" ("查询语句"), w6283, "'" ("字符串")) -> (w6296:string)
            n1185 = call "SQL_Select.vi"("要读取的列名"=string[] ["Last_Station", "Last_Result"], "表名"="Online", "error in (no error)"=w6288, "查询语句"=w6296, "查询条件"=TRUE, "connection reference"=w6289) -> ("error out"=w6287:errorcluster, "数据"=w6295:string[][])  [unwired: 3 in, 1 out]
            n1186 = case shown="错误" w6287 {
              tunnel: w6295 -> [w6307 _]
              tunnel: ["1" ("右扫码请求回复") "2" ("右扫码请求回复")] -> w6279
              tunnel: [TRUE TRUE] -> w6285
              tunnel: [w6301 w6308] -> w6282
              tunnel: [w6300 w6308] -> w6281
              frame No Error {
                n1187 = Index Array(array=w6307, index (row)=0 ("索引 (行)")) -> (element=w6304:string[])  [unwired: 1 in]
                n1188 = Index Array(array=w6304, index #1=0 ("索引 (行)")) -> (element #1=w6301:string, element #2=w6300:string)  [unwired: 1 in]
                "上一站号 (601)" <- w6301
                "上一站结果 (601)" <- w6300
              }
              frame Error {
                w6308 = ""
              }
            }
            "扫码请求回复601" <- w6279
            n1189 = Format Date/Time String(time format string (%c)="——%Y-%m-%d_%H-%M-%S" ("时间格式字符串(%c)")) -> (date/time string=w6278:string)  [unwired: 2 in]
            n1190 = local write "601扫码回复输入"(w6285) -> ()
            n1191 = Concatenate Strings(w6283, "——" ("字符串"), w6282, w6281, w6279, w6278) -> (w6277:string)
            n1192 = disable-structure shown="禁用" {
              disable-tunnel: w6277 -> [w6298 _]
              frame Disabled {
                n1193 = call "站点编码更新（年月日）.vi"("当前编码信息"=w6298, "站别"="601") -> ()  [unwired: 10 in]
              }
              frame Enabled {
              }
            }
            "ST601扫码请求（事件）" <- FALSE ("ST601扫码请求（事件）")
          }
          event "ST601数据读取（事件）": Value Change {
            w6333 = 0 ("索引 (行)")
            n1194 = event-data() -> ()  [unwired: 1 in, 2 out]
            n1195 = local read "601二维码"() -> (w6312:string)
            n1196 = Concatenate Strings("Where QRCode='" ("查询语句"), w6312, "'" ("字符串")) -> (w6340:string)
            n1197 = call "SQL_Select.vi"("要读取的列名"=string[] ["Rework_Status"], "表名"="Online", "error in (no error)"=w6326, "查询语句"=w6340, "查询条件"=TRUE, "connection reference"=w6327) -> ("error out"=w6335:errorcluster, "数据"=w6339:string[][], "connection reference out"=w6336:T5)  [unwired: 3 in]
            n1198 = Index Array(array=w6339, index (row)=w6333, index (col)=w6333) -> (element=w6338:string)
            n1199 = Equal?(x=w6338, y="T") -> (x = y?=w6337:bool)
            n1200 = local read "601数据"() -> (w6313:string[])
            n1201 = case shown="真" w6337 {
              tunnel: [w6354 w6360] -> w6324
              tunnel: w6313 -> [w6353 w6363]
              tunnel: [w6348 w6359] -> w6323
              tunnel: w6312 -> [w6347 w6362]
              tunnel: w6340 -> [w6346 w6361]
              tunnel: w6336 -> [w6345 w6374]
              tunnel: w6335 -> [w6344 w6373]
              tunnel: [TRUE w6358] -> w6325
              frame False {
                n1202 = call "SQL_Update.vi"("查询语句"=w6346, "表名"="Online", "error in (no error)"=w6344, "列名对应的值"=w6353, "列名"=string[] ["Last_Station", "Last_Result", "ST601_Date", "ST601_Time", "ST601_Result", "ST601_PanelNumber"], "connection reference"=w6345) -> ("error out"=w6348:errorcluster)  [unwired: 4 in, 1 out]
                n1203 = Unbundle By Name(w6348) -> ("status"=w6352:bool)
                n1204 = Equal?(x=w6347, y="") -> (x = y?=w6350:bool)
                n1205 = Or(x=w6352, y=w6350) -> (x .or. y?=w6349:bool)
                n1206 = case shown="假" w6349 {
                  tunnel: ["1" ("数据保存请求回复") "2" ("数据保存请求回复")] -> w6354
                  frame False {
                  }
                  frame True {
                  }
                }
              }
              frame True {
                w6369 = 0 ("索引 (行)")
                n1207 = call "SQL_Select.vi"("要读取的列名"=string[] ["[601]"], "表名"="Rework_List", "error in (no error)"=w6373, "查询语句"=w6361, "查询条件"=TRUE, "connection reference"=w6374) -> ("error out"=w6364:errorcluster, "数据"=w6370:string[][], "connection reference out"=w6365:T5)  [unwired: 3 in]
                n1208 = Index Array(array=w6370, index (row)=w6369, index (col)=w6369) -> (element=w6368:string)
                n1209 = Equal?(x=w6368, y="T") -> (x = y?=w6366:bool)
                n1210 = case shown="真" w6366 {
                  tunnel: w6365 -> [w6383 w6403]
                  tunnel: w6364 -> [w6384 w6402]
                  tunnel: w6363 -> [w6382 w6409]
                  tunnel: w6362 -> [w6379 w6404]
                  tunnel: w6361 -> [w6381 w6394]
                  tunnel: [w6378 w6396] -> w6360
                  tunnel: [w6380 w6395] -> w6359
                  tunnel: [TRUE TRUE] -> w6358
                  frame False {
                    n1211 = call "SQL_Update.vi"("查询语句"=w6381, "表名"="Online", "error in (no error)"=w6384, "列名对应的值"=w6382, "列名"=string[] ["Last_Station", "Last_Result", "ST601_Date", "ST601_Time", "ST601_Result", "ST601_PanelNumber"], "connection reference"=w6383) -> ("error out"=w6380:errorcluster)  [unwired: 4 in, 1 out]
                    n1212 = Unbundle By Name(w6380) -> ("status"=w6388:bool)
                    n1213 = Equal?(x=w6379, y="") -> (x = y?=w6386:bool)
                    n1214 = Or(x=w6388, y=w6386) -> (x .or. y?=w6385:bool)
                    n1215 = case shown="假" w6385 {
                      tunnel: ["1" ("数据保存请求回复") "2" ("数据保存请求回复")] -> w6378
                      frame False {
                      }
                      frame True {
                      }
                    }
                  }
                  frame True {
                    n1216 = Delete From Array(array=w6409, length=2 ("长度"), index=0 ("索引")) -> (deleted portion=w6397:string[], array with subset deleted=w6406:string[])
                    n1217 = call "SQL_Update.vi"("查询语句"=w6394, "表名"="Online", "error in (no error)"=w6402, "列名对应的值"=w6397, "列名"=string[] ["Last_Station", "Last_Result"], "connection reference"=w6403) -> ("error out"=w6401:errorcluster, "connection reference 2"=w6400:T5)  [unwired: 4 in]
                    n1218 = call "SQL_Update.vi"("查询语句"=w6394, "表名"="Rework", "error in (no error)"=w6401, "列名对应的值"=w6406, "列名"=string[] ["ST601_Date", "ST601_Time", "ST601_Result", "ST601_PanelNumber"], "connection reference"=w6400) -> ("error out"=w6395:errorcluster)  [unwired: 4 in, 1 out]
                    n1219 = Unbundle By Name(w6395) -> ("status"=w6412:bool)
                    n1220 = Equal?(x="", y=w6404) -> (x = y?=w6411:bool)
                    n1221 = Or(x=w6412, y=w6411) -> (x .or. y?=w6410:bool)
                    n1222 = case shown="真" w6410 {
                      tunnel: ["1" ("数据保存请求回复") "2" ("数据保存请求回复")] -> w6396
                      frame False {
                      }
                      frame True {
                      }
                    }
                  }
                }
              }
            }
            "数据保存请求回复601" <- w6324
            n1223 = Delete From Array(array=w6313, length=2 ("长度"), index=0 ("索引")) -> (array with subset deleted=w6320:string[])  [unwired: 1 out]
            n1224 = Insert Into Array(array=w6320, index=2 ("索引"), new element=w6312) -> (w6319:string[])
            n1225 = local write "601数据回复输入"(w6325) -> ()
            n1226 = Insert Into Array(array=string[][] [] ("数组"), index (row)=0 ("索引 (行)"), new element=w6319) -> (w6321:string[][])  [unwired: 1 in]
            n1227 = Transpose 2D Array(2D array=w6321) -> (transposed array=w6311:string[][])
            n1228 = property on="ST601_DATA" class="MCListbox (严格)"("ItemNames"=w6311) -> ()  [unwired: 2 in, 2 out]
            "ST601数据读取（事件）" <- FALSE ("ST601数据读取（事件）")
          }
          event "ST602扫码请求 （事件）": Value Change {
            n1229 = event-data() -> ()  [unwired: 1 in, 2 out]
            n1230 = local read "602二维码"() -> (w6420:string)
            n1231 = Concatenate Strings("Where QRCode='" ("查询语句"), w6420, "'" ("字符串")) -> (w6429:string)
            n1232 = call "SQL_Select.vi"("要读取的列名"=string[] ["Last_Station", "Last_Result"], "表名"="Online", "error in (no error)"=w6421, "查询语句"=w6429, "查询条件"=TRUE, "connection reference"=w6422) -> ("error out"=w6419:errorcluster, "数据"=w6428:string[][])  [unwired: 3 in, 1 out]
            n1233 = case shown="无错误" w6419 {
              tunnel: w6428 -> [w6438 _]
              tunnel: ["1" ("右扫码请求回复") "2" ("右扫码请求回复")] -> w6417
              tunnel: [TRUE TRUE] -> w6416
              frame No Error {
                n1234 = Index Array(array=w6438, index (row)=0 ("索引 (行)")) -> (element=w6435:string[])  [unwired: 1 in]
                n1235 = Index Array(array=w6435, index #1=0 ("索引 (行)")) -> (element #1=→"上一站号 (602)":string, element #2=→"上一站结果 (602)":string)  [unwired: 1 in]
              }
              frame Error {
              }
            }
            "扫码请求回复602" <- w6417
            n1236 = local write "602扫码回复输入"(w6416) -> ()
            "ST602扫码请求 （事件）" <- FALSE ("ST602扫码请求 （事件）")
          }
          event "ST602数据读取（事件）": Value Change {
            w6463 = 0 ("索引 (行)")
            n1237 = event-data() -> ()  [unwired: 1 in, 2 out]
            n1238 = local read "602二维码"() -> (w6442:string)
            n1239 = Concatenate Strings("Where QRCode='" ("查询语句"), w6442, "'" ("字符串")) -> (w6470:string)
            n1240 = call "SQL_Select.vi"("要读取的列名"=string[] ["Rework_Status"], "表名"="Online", "error in (no error)"=w6456, "查询语句"=w6470, "查询条件"=TRUE, "connection reference"=w6457) -> ("error out"=w6465:errorcluster, "数据"=w6469:string[][], "connection reference out"=w6466:T5)  [unwired: 3 in]
            n1241 = Index Array(array=w6469, index (row)=w6463, index (col)=w6463) -> (element=w6468:string)
            n1242 = Equal?(x=w6468, y="T") -> (x = y?=w6467:bool)
            n1243 = local read "602data"() -> (w6443:string[])
            n1244 = case shown="真" w6467 {
              tunnel: [w6484 w6490] -> w6455
              tunnel: w6443 -> [w6483 w6493]
              tunnel: [w6478 w6489] -> w6453
              tunnel: w6442 -> [w6477 w6492]
              tunnel: w6470 -> [w6476 w6491]
              tunnel: w6466 -> [w6475 w6504]
              tunnel: w6465 -> [w6474 w6503]
              tunnel: [TRUE w6488] -> w6454
              frame False {
                n1245 = call "SQL_Update.vi"("查询语句"=w6476, "表名"="Online", "error in (no error)"=w6474, "列名对应的值"=w6483, "列名"=string[] ["Last_Station", "Last_Result", "ST602_Date", "ST602_Time", "ST602_Result", "ST602_PanelNumber"], "connection reference"=w6475) -> ("error out"=w6478:errorcluster)  [unwired: 4 in, 1 out]
                n1246 = Unbundle By Name(w6478) -> ("status"=w6482:bool)
                n1247 = Equal?(x=w6477, y="") -> (x = y?=w6480:bool)
                n1248 = Or(x=w6482, y=w6480) -> (x .or. y?=w6479:bool)
                n1249 = case shown="假" w6479 {
                  tunnel: ["1" ("数据保存请求回复") "2" ("数据保存请求回复")] -> w6484
                  frame False {
                  }
                  frame True {
                  }
                }
              }
              frame True {
                w6499 = 0 ("索引 (行)")
                n1250 = call "SQL_Select.vi"("要读取的列名"=string[] ["[602]"], "表名"="Rework_List", "error in (no error)"=w6503, "查询语句"=w6491, "查询条件"=TRUE, "connection reference"=w6504) -> ("error out"=w6494:errorcluster, "数据"=w6500:string[][], "connection reference out"=w6495:T5)  [unwired: 3 in]
                n1251 = Index Array(array=w6500, index (row)=w6499, index (col)=w6499) -> (element=w6498:string)
                n1252 = Equal?(x=w6498, y="T") -> (x = y?=w6496:bool)
                n1253 = case shown="真" w6496 {
                  tunnel: w6495 -> [w6513 w6533]
                  tunnel: w6494 -> [w6514 w6532]
                  tunnel: w6493 -> [w6512 w6539]
                  tunnel: w6492 -> [w6509 w6534]
                  tunnel: w6491 -> [w6511 w6524]
                  tunnel: [w6508 w6526] -> w6490
                  tunnel: [w6510 w6525] -> w6489
                  tunnel: [TRUE TRUE] -> w6488
                  frame False {
